vi "FGV Image.vi"(7 "CMD":T2, 8 "error in (no error)":errorcluster, 11 "Image In":T1) -> (0 "error out":errorcluster, 3 "Image Out":T1)   [LabVIEW 2020]
uses:
  PCT FGV CMD.ctl
  <vilib>/vision/Image Controls.llb/IMAQ Image.ctl
panel:
  # "0 - Gage at Zero\n1 - GF"
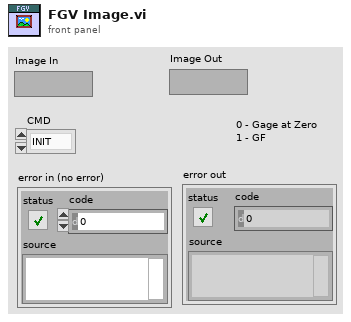
[diagram p1: front panel]
types:
  T1 = typedef "IMAQ Image.ctl" = refnum<image>
  T2 = typedef "PCT FGV CMD.ctl" = enum16{"INIT", "GET", "SET"}
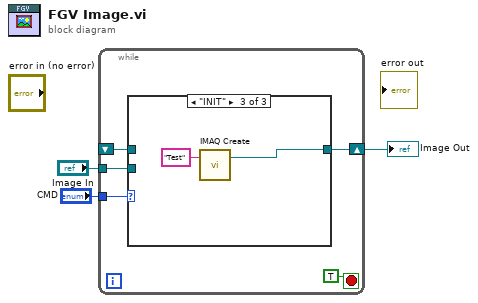
[diagram p0: block diagram]
diagram:
  n1 = while {
    tunnel: "Image In" -> [w6]
    tunnel: "CMD" -> [w8]
    shift-right: [w5] -> w3
    shift-left: _ -> [w7]
    stop <- TRUE stop-if-true
    n2 = case shown="\"INIT\"" w8 {
      tunnel: w7 -> [_ w10 _]
      tunnel: w6 -> [w9 _ _]
      tunnel: [w9 w10 w12] -> w5
      frame "SET", Default {
      }
      frame "GET" {
      }
      frame "INIT" {
        n3 = call "IMAQ Create"("Image Name"="Test") -> ("New Image"=w12:T1)  [unwired: 3 in, 2 out]
      }
    }
  }
  "Image Out" <- w3
